vi "Set Server State Ref.vi"(10 "Server Internal State Ref":refnum<data-value>, 11 "Template Server in":refnum<class "ctet_dio.lvclass">) -> (3 "Template Server out":refnum<class "ctet_dio.lvclass">)   [LabVIEW 2019, in "ctet_dio.lvlib" / "ctet_dio.lvclass"]
uses:
  ctet_dio.lvclass
  typeDefs/Server State Data.ctl
  ctet_dio.lvclass/ctet_dio.ctl
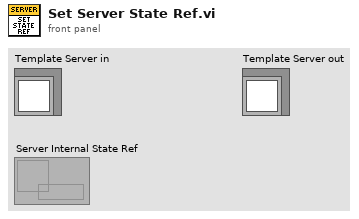
[diagram p1: front panel]
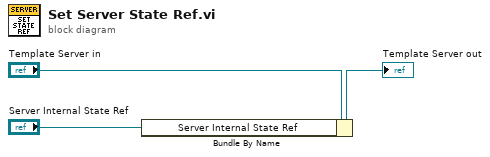
[diagram p0: block diagram]
diagram:
  n1 = Bundle By Name(cluster="Template Server in", "Server Internal State Ref"="Server Internal State Ref") -> (→"Template Server out":refnum<class "ctet_dio.lvclass">)
